vi "Keep true until....vi"(1 "Changer":bool, 2 "Keep":bool) -> (0 "Value":bool)   [LabVIEW 2012]
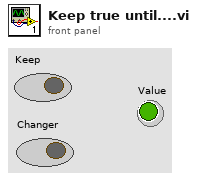
[diagram p1: front panel]
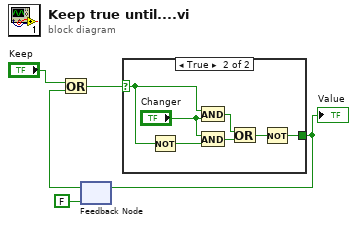
[diagram p0: block diagram]
diagram:
  n1 = feedback #1(FALSE) -> (w2:bool)
  n2 = Or(x="Keep", y=w2) -> (x .or. y?=w3:bool)
  n3 = case shown="True" w3 {
    selector: w3 -> [w6 w8]
    tunnel: [w6 w7] -> w1
    frame False {
    }
    frame True {
      n4 = Not(x=w8) -> (.not. x?=w9:bool)
      n5 = And(x=w8, y="Changer") -> (x .and. y?=w11:bool)
      n6 = And(x="Changer", y=w9) -> (x .and. y?=w12:bool)
      n7 = Or(x=w11, y=w12) -> (x .or. y?=w13:bool)
      n8 = Not(x=w13) -> (.not. x?=w7:bool)
    }
  }
  "Value" <- w1
  n9 = feedback-in #1(w1) -> ()
